vi "JSONToMeasurementConfig.vi"(8 "ErrorIn":errorcluster, 11 "JSONIn":refnum<class "JSON Value.lvclass">) -> (0 "ErrorOut":errorcluster, 2 "MeasurementConfig":T1={"Frequency"=100, "Resolution[b]"=16, "AccelFSRange"=enum."+/-2g", "GyroFSRange"=enum."+/-250dps"} {"Resolution[b]" min=4 max=16 step=1; "Frequency" min=1 max=10000000 step=1}, 3 "JSONOut":refnum<class "JSON Value.lvclass">)   [LabVIEW 2016]
doc: "Convert JSON to MeasurementConfig."
uses:
  FallSensor/MeasurementConfig.ctl
  FallSensor/Measurement/AccelFSRange.ctl
  FallSensor/Measurement/GyroFSRange.ctl
  <vilib>/addons/JSON API/JSON Value/JSON Value.lvclass
  <vilib>/addons/JSON API/JSON Value/Get Object Item by Name.vi
  <vilib>/addons/JSON API/JSON Scalar/Get as U32.vi
  <vilib>/addons/JSON API/Get Polymorphic/JSON GetSet.lvlib
  <vilib>/addons/JSON API/JSON Scalar/JSON Scalar.lvclass
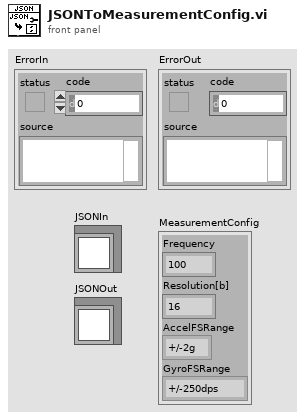
[diagram p1: front panel]
types:
  T1 = typedef "MeasurementConfig.ctl" = cluster{"Frequency":u32, "Resolution[b]":u32, "AccelFSRange":T2, "GyroFSRange":T3}
  T2 = typedef "AccelFSRange.ctl" = enum16{"+/-2g", "+/-4g", "+/-8g", "+/-16g"}
  T3 = typedef "GyroFSRange.ctl" = enum16{"+/-250dps", "+/-500dps", "+/-1000dps", "+/-2000dps"}
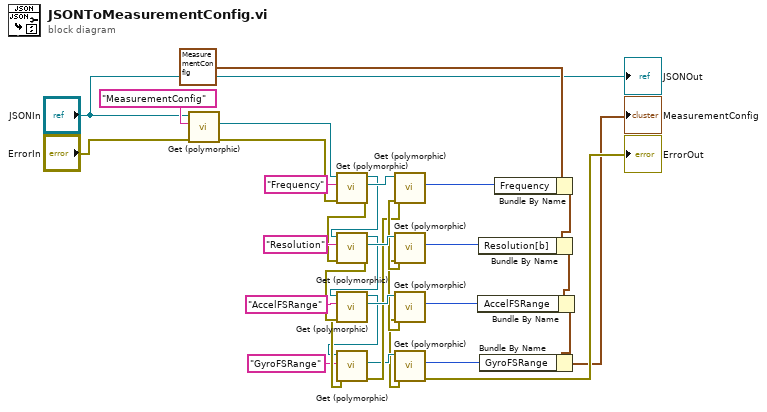
[diagram p0: block diagram]
diagram:
  n1 = call-poly <vilib>:"Get (polymorphic).vi"("error in (no error)"="ErrorIn", "name"="MeasurementConfig", "JSON Value In"="JSONIn") -> ("error out"=w4:errorcluster, "Value"=w3:refnum<class "JSON Value.lvclass">)  [unwired: 5 in, 2 out]
  n2 = call-poly <vilib>:"Get (polymorphic).vi"("error in (no error)"=w4, "name"="Frequency", "JSON Value In"=w3) -> ("error out"=w25:errorcluster, "Value"=w32:refnum<class "JSON Value.lvclass">, "JSON Value Out"=w29:refnum<class "JSON Value.lvclass">)  [unwired: 5 in, 1 out]
  n3 = call-poly <vilib>:"Get (polymorphic).vi"("error in (no error)"=w25, "name"="Resolution", "JSON Value In"=w29) -> ("error out"=w24:errorcluster, "Value"=w28:refnum<class "JSON Value.lvclass">, "JSON Value Out"=w27:refnum<class "JSON Value.lvclass">)  [unwired: 5 in, 1 out]
  n4 = call-poly <vilib>:"Get (polymorphic).vi"("error in (no error)"=w24, "name"="AccelFSRange", "JSON Value In"=w27) -> ("error out"=w18:errorcluster, "Value"=w26:refnum<class "JSON Value.lvclass">, "JSON Value Out"=w14:refnum<class "JSON Value.lvclass">)  [unwired: 5 in, 1 out]
  n5 = call-poly <vilib>:"Get (polymorphic).vi"("error in (no error)"=w18, "name"="GyroFSRange", "JSON Value In"=w14) -> ("error out"=w16:errorcluster, "Value"=w15:refnum<class "JSON Value.lvclass">)  [unwired: 5 in, 2 out]
  n6 = call-poly <vilib>:"Get (polymorphic).vi"("error in (no error)"=w16, "JSON Scalar in"=w32) -> ("error out"=w23:errorcluster, "Number"=w21:u32)  [unwired: 7 in, 1 out]
  n7 = call-poly <vilib>:"Get (polymorphic).vi"("error in (no error)"=w23, "JSON Scalar in"=w28) -> ("error out"=w22:errorcluster, "Number"=w19:u32)  [unwired: 7 in, 1 out]
  n8 = call-poly <vilib>:"Get (polymorphic).vi"("error in (no error)"=w22, "JSON Scalar in"=w26) -> ("error out"=w13:errorcluster, "Number"=w7:u32)  [unwired: 7 in, 1 out]
  n9 = call-poly <vilib>:"Get (polymorphic).vi"("error in (no error)"=w13, "JSON Scalar in"=w15) -> ("error out"=→"ErrorOut":errorcluster, "Number"=w9:u32)  [unwired: 7 in, 1 out]
  n10 = Bundle By Name(cluster=T1 {"Frequency"=100, "Resolution[b]"=16, "AccelFSRange"=enum."+/-2g", "GyroFSRange"=enum."+/-250dps"} ("MeasurementConfig 2"), "Frequency"=w21) -> (w20:T1)
  n11 = Bundle By Name(cluster=w20, "Resolution[b]"=w19) -> (w10:T1)
  n12 = Bundle By Name(cluster=w10, "AccelFSRange"=w7) -> (w8:T1)
  n13 = Bundle By Name(cluster=w8, "GyroFSRange"=w9) -> (→"MeasurementConfig":T1)
  "JSONOut" <- "JSONIn"
